vi "add_Transform.vi"(6 "Transform":T1, 7 "msg in":string) -> (3 "msg out":string)   [LabVIEW 2012]
doc: "Flattens a transform into a message"
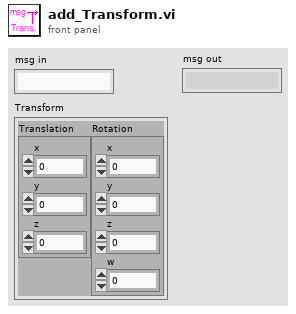
[diagram p1: front panel]
types:
  T1 = cluster{"Translation":cluster{"x":dbl, "y":dbl, "z":dbl}, "Rotation":cluster{"x":dbl, "y":dbl, "z":dbl, "w":dbl}}
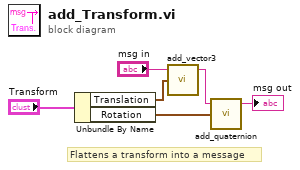
[diagram p0: block diagram]
diagram:
  # "Flattens a transform into a message"
  n1 = Unbundle By Name("Transform") -> ("Translation"=w2:cluster{"x":dbl, "y":dbl, "z":dbl}, "Rotation"=w1:cluster{"x":dbl, "y":dbl, "z":dbl, "w":dbl})
  n2 = call "add_vector3.vi"("Vector3"=w2, "msg in"="msg in") -> ("msg out"=w5:string)  [unwired: 3 in]
  n3 = call "add_quaternion.vi"("Quaternion"=w1, "msg in"=w5) -> ("msg out"=→"msg out":string)  [unwired: 3 in]
